vi "Config Sample Scan.vi"(6 "Delta (1)":i32(ring)=1 items=["-1"=-1, "1"=1], 7 "Coupling (0)":i32 min=0 max=3, 8 "error in":errorcluster, 9 "Ceiling (8)":i32=8 min=1 max=8, 10 "Floor (1)":i32=1 min=1 max=8, 11 "VISA resource name":refnum<visa-resource-name>) -> (0 "error out":errorcluster, 3 "VISA resource name out":refnum<visa-resource-name>)   [LabVIEW 2014, in "Andeen-Hagerling 2700.lvlib"]
doc: "This VI establishes the position of sample switch scanning within the multidimensional parameter scanning system. Also sets the highest and lowest sample switch numbers to be used during scanning. and the direction in which the sample number is changed each time a scan measurement is to be taken."
uses:
  Andeen-Hagerling 2700.lvlib
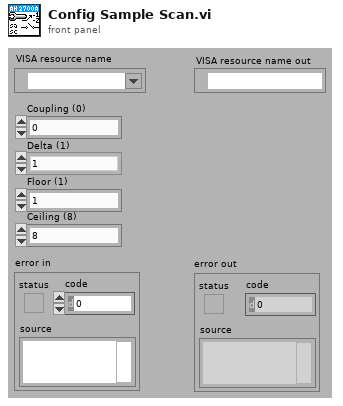
[diagram p1: front panel]
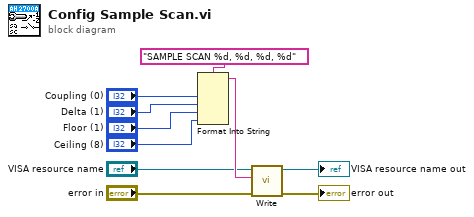
[diagram p0: block diagram]
diagram:
  n1 = Format Into String(format string="SAMPLE SCAN %d, %d, %d, %d", "Coupling (0)", "Delta (1)", "Floor (1)", "Ceiling (8)") -> (resulting string=w7:string)  [unwired: 2 in, 1 out]
  n2 = call "Write.vi"("error in"="error in", "command"=w7, "VISA resource name"="VISA resource name") -> ("error out"=→"error out":errorcluster, "VISA resource name out"=→"VISA resource name out":refnum<visa-resource-name>)  [unwired: 7 in]
